vi "2100_Compare Expected and Actual Reg Info.vi"(9 "Readback_Array":T1[](array[typedef]) {"Address" format="%.0x"}, 11 "Master_Register_Data_Array_In":T2=[{"Address"=6, "Data"=1}, {"Address"=7, "Data"=2}, {"Address"=8, "Data"=3}] {"Address" format="%.0x"}) -> (2 "Readback_Values":u8[](array[numeric]), 3 "Trim_Read_Fail":i16)   [LabVIEW 2013]
uses:
  Controls/Master_Reg_Data_Array.ctl
  Controls/Reg_Address_Data.ctl
panel:
  out "Trim_Read_Match":bool
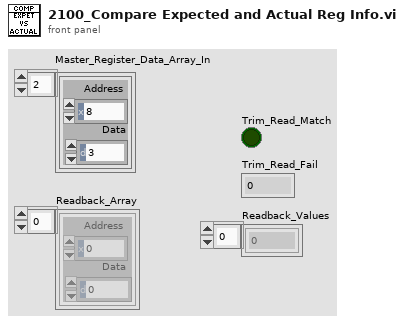
[diagram p1: front panel]
types:
  T1 = typedef "Reg_Address_Data.ctl" = cluster{"Address":u8, "Data":u8}
  T2 = typedef "Master_Reg_Data_Array.ctl" = T1[]
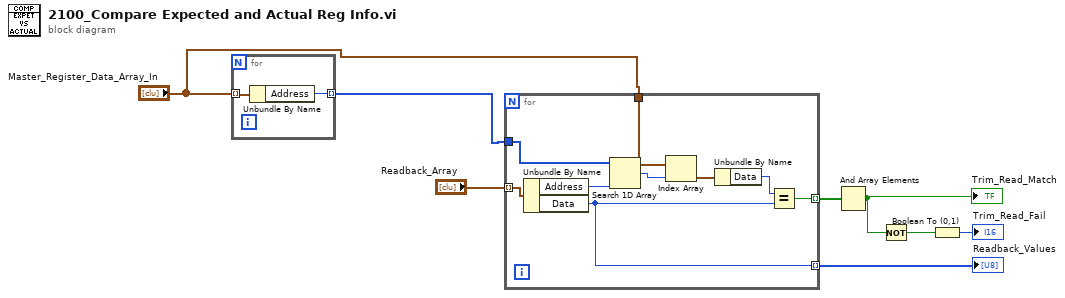
[diagram p0: block diagram]
diagram:
  n1 = for {
    tunnel: "Master_Register_Data_Array_In" -> [w10] mode=indexing
    tunnel: [w9] -> w4 mode=indexing
    n2 = Unbundle By Name(w10) -> ("Address"=w9:u8)
  }
  n3 = for {
    tunnel: "Readback_Array" -> [w19] mode=indexing
    tunnel: w4 -> [w18]
    tunnel: "Master_Register_Data_Array_In" -> [w16]
    tunnel: [w12] -> w2 mode=indexing
    tunnel: [w11] -> w1 mode=indexing
    n4 = Unbundle By Name(w19) -> ("Address"=w17:u8, "Data"=w11:u8)
    n5 = Search 1D Array(1D array=w18, element=w17) -> (index of element=w15:i32)  [unwired: 1 in]
    n6 = Index Array(array=w16, index=w15) -> (element=w14:T1)
    n7 = Unbundle By Name(w14) -> ("Data"=w13:u8)
    n8 = Equal?(x=w13, y=w11) -> (x = y?=w12:bool)
  }
  "Readback_Values" <- w1
  n9 = And Array Elements(Boolean array=w2) -> (logical AND=w7:bool)
  "Trim_Read_Match" <- w7
  n10 = Not(x=w7) -> (.not. x?=w6:bool)
  n11 = Boolean To (0,1)(Boolean=w6) -> (0, 1=→"Trim_Read_Fail":i16)
